vi "TTA_Update_Test_Status_Refnum.vi"(8 "error in":errorcluster, 11 "Test Status Refnum":refnum<vi>) -> (0 "error out":errorcluster)   [LabVIEW 2016]
uses:
  TTA_Globals/Test_Status.vi
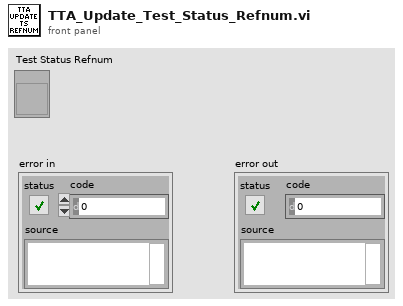
[diagram p1: front panel]
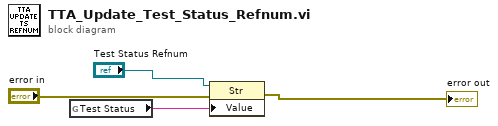
[diagram p0: block diagram]
diagram:
  n1 = global read "Test_Status.vi" "Test Status"() -> (w3:string)
  n2 = property class="Str"(reference="Test Status Refnum", error in="error in", "Value"=w3) -> (error out=→"error out":errorcluster)  [unwired: 1 out]
